vi "backup_nvm.vi"(6 "timeout (25000ms)":i32=25000, 8 "error in (no error)":errorcluster, 9 "type":T1, 10 "File Path":path, 11 "daemon reference in":refnum<k5>) -> (0 "error out":errorcluster, 2 "response":string, 3 "daemon reference out":refnum<k5>, 5 "command out":string="random")   [LabVIEW 2017]
doc: "<b>Command: </b>\"backup_nvm\"\n\n<b>Description: </b>Queries the 683 and backs up the nvm data to a file in json file format that can be used to restore the nvm if necessary.\n\n<b>Note: </b>This command can take up to 10 seconds to capture the nvm data.\n____________________________________________\nDIPC 692 Daemon API 10.0.0.1\nSam Tee - Dyson Technology Ltd\nCopyright (c) 2024, Dyson Technology Ltd"
uses:
  typdef/read_nvm_section.ctl
panel:
  # "input the filename in .json format"
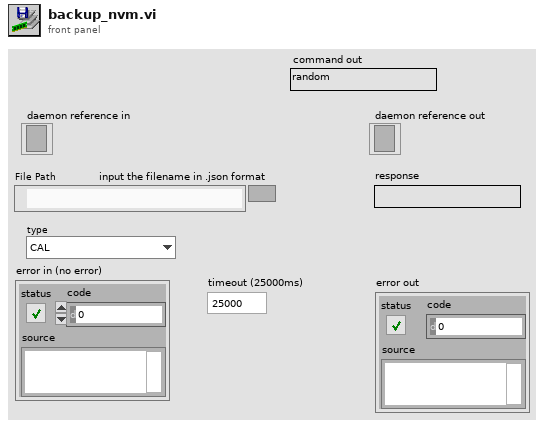
[diagram p1: front panel]
types:
  T1 = typedef "read_nvm_section.ctl" = enum16{"CAL", "ERROR", "USAGE"}
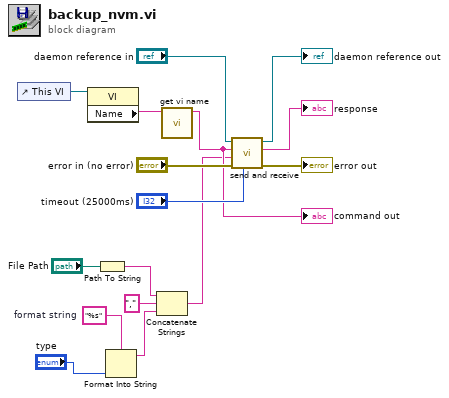
[diagram p0: block diagram]
diagram:
  w4 = "%s"  # format string
  n1 = control-ref of="This VI"() -> (w10:refnum<vi>)
  n2 = property class="VI"(reference=w10) -> ("Name"=w9:string)  [unwired: 1 in, 2 out]
  n3 = Path To String(path="File Path") -> (string=w6:string)
  n4 = Format Into String(format string=w4, "type") -> (resulting string=w2:string)  [unwired: 2 in, 1 out]
  n5 = Concatenate Strings(w6, "," ("string"), w2) -> (w1:string)
  n6 = call "get vi name.vi"("library.lvlib:name.vi"=w9) -> ("vi name"=w8:string)  [unwired: 10 in]
  "command out" <- w8
  n7 = call "send and receive.vi"("timeout (25000ms)"="timeout (25000ms)", "error in (no error)"="error in (no error)", "data"=w1, "command"=w8, "daemon reference in"="daemon reference in") -> ("error out"=→"error out":errorcluster, "response"=→"response":string, "daemon reference out"=→"daemon reference out":refnum<k5>)  [unwired: 4 in]
